vi "Set Region.vi"(8 "error in (no error)":errorcluster, 9 "Image Size":T1, 10 "Image Offset":T2, 11 "Camera in":refnum<class "Camera.lvclass">) -> (0 "error out":errorcluster, 3 "Camera":refnum<class "Camera.lvclass">)   [LabVIEW 2020, in "Camera.lvclass"]
uses:
  Camera.lvclass
  Camera.lvclass/Camera.ctl
  Image Offset.ctl
  Buffer/Image Size.ctl
  Buffer/Buffer.lvclass
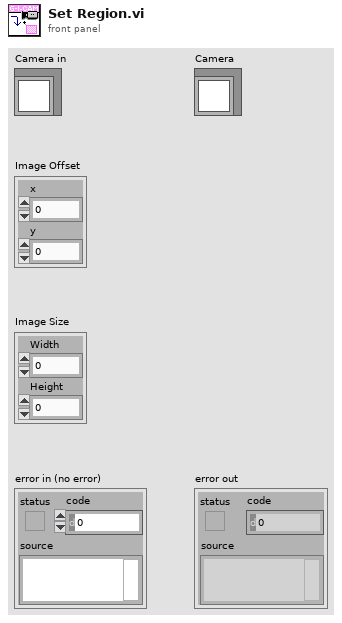
[diagram p1: front panel]
types:
  T1 = typedef "Buffer.lvclass/Image Size.ctl" = cluster{"Width":u16, "Height":u16}
  T2 = typedef "Camera.lvclass/Image Offset.ctl" = cluster{"x":i32, "y":i32}
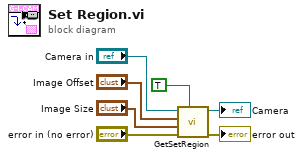
[diagram p0: block diagram]
diagram:
  n1 = call "GetSetRegion.vi"("Set"=TRUE, "error in (no error)"="error in (no error)", "Image Size"="Image Size", "Image Offset"="Image Offset", "Camera in"="Camera in") -> ("error out"=→"error out":errorcluster, "Camera"=→"Camera":refnum<class "Camera.lvclass">)  [unwired: 3 in, 2 out]
